vi "GetCtlRef_Lookup.vi"(8 "Error in":errorcluster, 10 "CtlName In":string, 11 "CtlLookup In":T1) -> (0 "error out":errorcluster, 1 "CtlRef":refnum<vi>, 2 "CtlName Out":string, 3 "CtlLookup Out":T1, 4 "Control Label Found?":bool)   [LabVIEW 2018, in "CtlReferences.lvlib" / "CtlReferences.lvclass"]
uses:
  CtlReferences.lvclass
  TypeDefs/CtlLookup.ctl
  CtlReferences.lvclass/CtlReferences.ctl
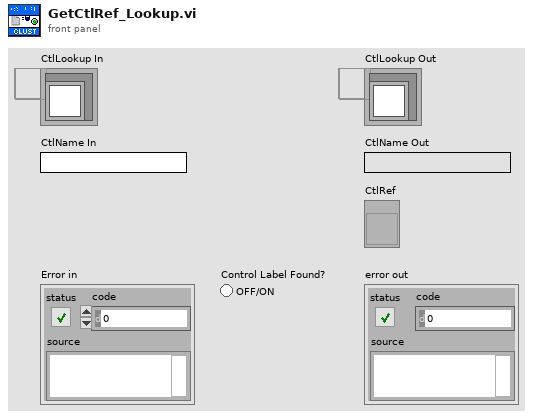
[diagram p1: front panel]
types:
  T1 = typedef "CtlReferences.lvlib/CtlReferences.lvclass/CtlLookup.ctl" = refnum<data-value>
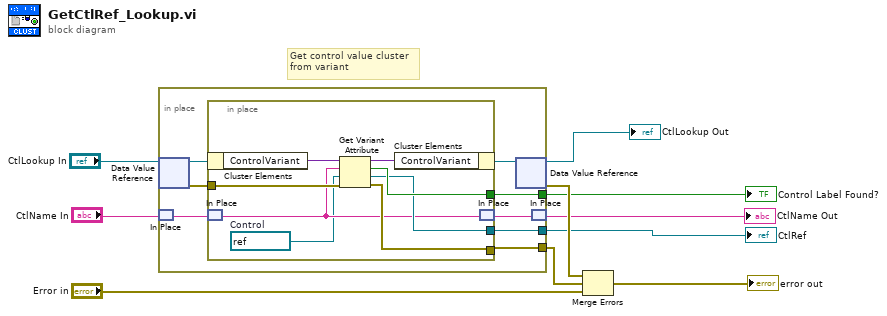
[diagram p0: block diagram]
diagram:
  # "Get control value cluster\nfrom variant"
  n1 = in-place {
    in-place-border: [w17] -> w7
    in-place-border: [w16] -> w10
    in-place-border: [w15] -> w1
    n2 = in-place-dvr #1("CtlLookup In") -> (w14:refnum<class "CtlReferences.lvclass">, w18:errorcluster)
    n3 = in-place-match #2("CtlName In") -> (w12:string)
    n4 = in-place {
      in-place-border: w18 -> [w26]
      in-place-border: [w25] -> w17
      in-place-border: [w24] -> w16
      in-place-border: [w21] -> w15
      w19 = refnum<vi> refnum  # Control
      n5 = in-place-cluster #3(w14) -> ("ControlVariant"=w23:variant)
      n6 = in-place-match #4(w12) -> (w20:string)
      n7 = Get Variant Attribute(Variant=w23, name=w20, default value (empty Variant)=w19, error in=w26) -> (duplicate Variant=w22:variant, found=w25:bool, value=w21:refnum<vi>, error out=w24:errorcluster)
      n8 = in-place-cluster #3("ControlVariant"=w22) -> (w13:refnum<class "CtlReferences.lvclass">)
      n9 = in-place-match #4(w20) -> (w11:string)
    }
    n10 = in-place-dvr #1(w13) -> (→"CtlLookup Out":T1, w9:errorcluster)
    n11 = in-place-match #2(w11) -> (→"CtlName Out":string)
  }
  "Control Label Found?" <- w7
  "CtlRef" <- w1
  n12 = Merge Errors(w9, w10, "Error in") -> (→"error out":errorcluster)
